vi "startUI.vi"(8 "error in (no error)":errorcluster, 10 "AMC*":T1, 11 "xceDataNode in":refnum<class "xceDataNode.lvclass">) -> (0 "error out":errorcluster, 2 "UI VI*":refnum<vi>, 3 "xceDataNode out":refnum<class "xceDataNode.lvclass">)   [LabVIEW 2013, in "xceDataNode.lvclass"]
doc: "Starts the user interface VI for this xceDataNode. This is the precursor to loading the UI VI into the xceSubpanel class. Also this VI is dynamic dispatch because it is just the suggested way to start a dynamic VI. This has been created with the idea that your classes UI VI will be created from the DataNodeUI.vit template."
uses:
  xceDataNode.lvclass
  <vilib>/NI/AMC/Message Queue.ctl
  <vilib>/NI/AMC/Message.ctl
  <vilib>/NI/Tools/Keyed Array/KeyedArray.ctl
  xceDataNode.lvclass/xceDataNode.ctl
  xceNode/xceNode.lvclass
  <vilib>/NI/AMC/AMC.lvlib
  <vilib>/NI/Tools/Keyed Array/Tools_KeyedArray.lvlib
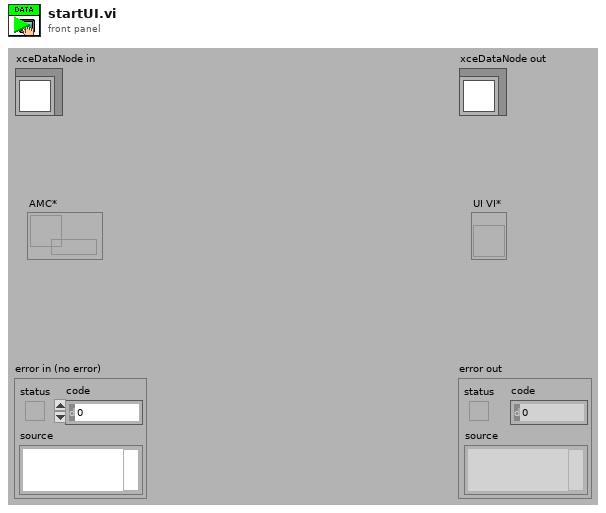
[diagram p1: front panel]
types:
  T1 = typedef "AMC.lvlib/Message Queue.ctl" = refnum<queue>
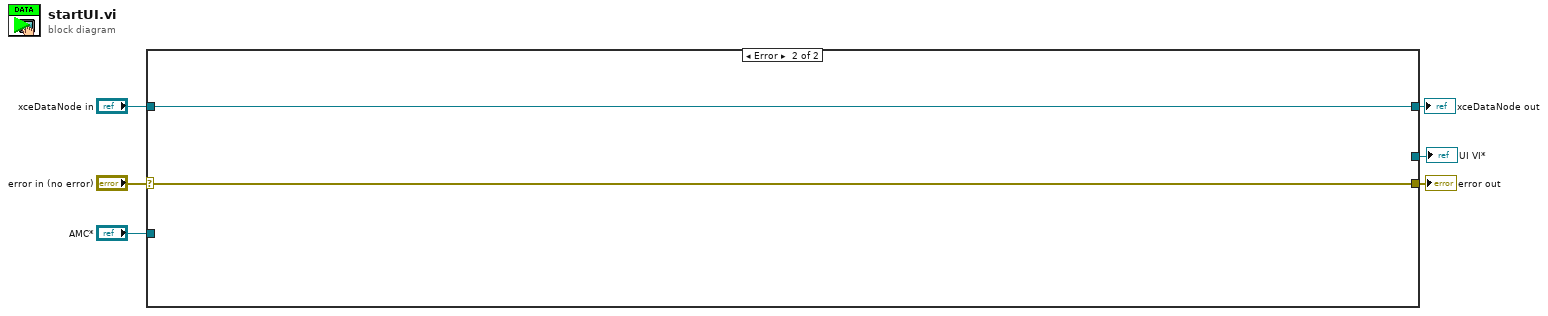
[diagram p0: block diagram]
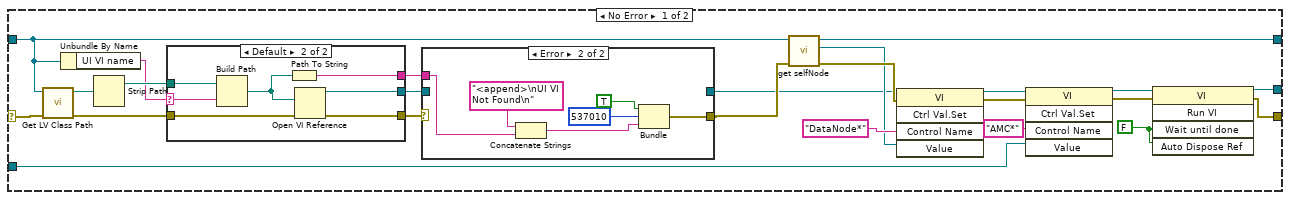
[diagram p2: hidden frame]
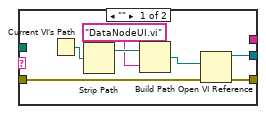
[diagram p3: hidden frame]
diagram:
  n1 = case shown="Error" "error in (no error)" {
    selector: "error in (no error)" -> [w16 w54]
    tunnel: [w21 w54] -> w5
    tunnel: [w29 w53] -> w3
    tunnel: "xceDataNode in" -> [w15 w53]
    tunnel: "AMC*" -> [w25 _]
    tunnel: [w20 _] -> w1
    frame No Error {
      w22 = FALSE ("Wait Until Done")
      n2 = call <vilib>:"Get LV Class Path.vi"("error in (no error)"=w16, "object"=w15) -> ("error out"=w13:errorcluster, "class path"=w17:path)  [unwired: 8 in]
      n3 = Unbundle By Name(w15) -> ("UI VI name"=w8:string)
      n4 = Strip Path(path=w17) -> (stripped path=w14:path)  [unwired: 1 out]
      n5 = case shown="Default" w8 {
        selector: w8 -> [_ w40]
        tunnel: w14 -> [_ w44]
        tunnel: w13 -> [w31 w43]
        tunnel: [w32 w42] -> w12
        tunnel: [w33 w41] -> w11
        tunnel: [_ w38] -> w7
        frame "" {
          n6 = Current VI's Path() -> (path=w35:path)
          n7 = Strip Path(path=w35) -> (stripped path=w36:path)  [unwired: 1 out]
          n8 = Build Path(base path=w36, name or relative path="DataNodeUI.vi") -> (appended path=w37:path)
          n9 = Open VI Reference(vi path=w37, error in (no error)=w31) -> (vi reference=w33:refnum<vi>, error out=w32:errorcluster)  [unwired: 4 in]
        }
        frame Default {
          n10 = Build Path(base path=w44, name or relative path=w40) -> (appended path=w39:path)
          n11 = Path To String(path=w39) -> (string=w38:string)
          n12 = Open VI Reference(vi path=w39, error in (no error)=w43) -> (vi reference=w41:refnum<vi>, error out=w42:errorcluster)  [unwired: 4 in]
        }
      }
      n13 = case shown="Error" w12 {
        selector: w12 -> [w46 _]
        tunnel: [w45 _] -> w9
        tunnel: [w46 w48] -> w10
        tunnel: w11 -> [w45 _]
        tunnel: w7 -> [_ w47]
        frame No Error {
        }
        frame Error {
          n14 = Concatenate Strings("<append>\nUI VI Not Found\n" ("source"), w47) -> (w51:string)
          n15 = Bundle("status"=TRUE, "code"=537010, w51) -> (w48:cluster{"status":bool, "code":i32, string})  [unwired: 1 out]
        }
      }
      n16 = call "get selfNode.vi"("error in (no error)"=w10, "xceNode in"=w15) -> ("error out"=w19:errorcluster, "selfNode*"=w18:refnum<data-value>, "xceNode out"=w29:refnum<class "xceDataNode.lvclass">)  [unwired: 7 in]
      n17 = invoke class="VI" method="Ctrl Val.Set"(reference=w9, error in=w19, "Control Name"="DataNode*", "Value"=w18) -> (reference out=w28:refnum<vi>, error out=w27:errorcluster)  [unwired: 1 in, 3 out]
      n18 = invoke class="VI" method="Ctrl Val.Set"(reference=w28, error in=w27, "Control Name"="AMC*", "Value"=w25) -> (reference out=w24:refnum<vi>, error out=w23:errorcluster)  [unwired: 1 in, 3 out]
      n19 = invoke class="VI" method="Run VI"(reference=w24, error in=w23, "Wait until done"=w22, "Auto Dispose Ref"=w22) -> (reference out=w20:refnum<vi>, error out=w21:errorcluster)  [unwired: 1 in, 3 out]
    }
    frame Error {
    }
  }
  "error out" <- w5
  "xceDataNode out" <- w3
  "UI VI*" <- w1
